vi "FGV Messbetrieb.vi"(0 "messen":bool, 11 "error in (no error)":errorcluster caption="Fehler (Eingang, kein Fehler)", 13 "Aktion":T1) -> (4 "messen":bool, 15 "error out":errorcluster caption="Fehler (Ausgang)")   [LabVIEW 2020, in "Allgemein.lvlib"]
uses:
  Allgemein.lvlib
  Aktion FGV Messbetrieb.ctl
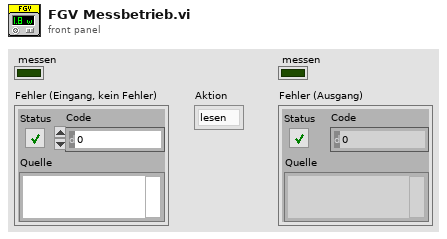
[diagram p1: front panel]
types:
  T1 = typedef "Allgemein.lvlib/Aktion FGV Messbetrieb.ctl" = enum16{"lesen", "schreiben"}
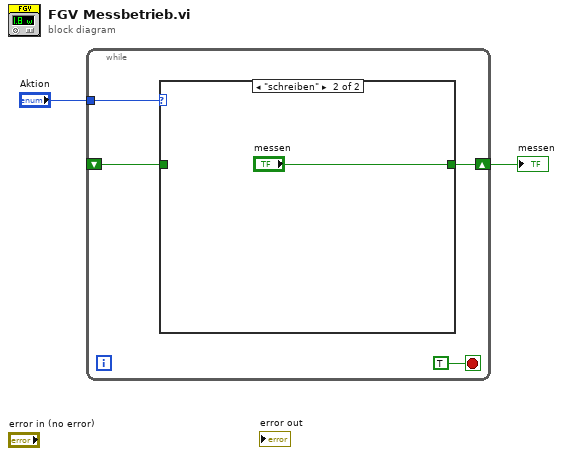
[diagram p0: block diagram]
diagram:
  n1 = while {
    tunnel: "Aktion" -> [w5]
    shift-right: [w4] -> w1
    shift-left: _ -> [w3]
    stop <- TRUE stop-if-true
    n2 = case shown="\"schreiben\"" w5 {
      tunnel: [w7 "messen"] -> w4
      tunnel: w3 -> [w7 _]
      frame "lesen", Default {
      }
      frame "schreiben" {
      }
    }
  }
  "messen" <- w1
